vi "parseEngineeringStatus.vi"(8 "error in (no error)":errorcluster, 10 "engineeringStatusString":string, 11 "DomeCommunicator in":refnum<class "DomeCommunicator.lvclass">) -> (0 "error out":errorcluster, 2 "engineeringStatus":T1, 3 "DomeCommunicator out":refnum<class "DomeCommunicator.lvclass">)   [LabVIEW 2016, in "DomeCommunicator.lvclass"]
uses:
  DomeCommunicator.lvclass
  ComTypedefs/engineeringStatus.ctl
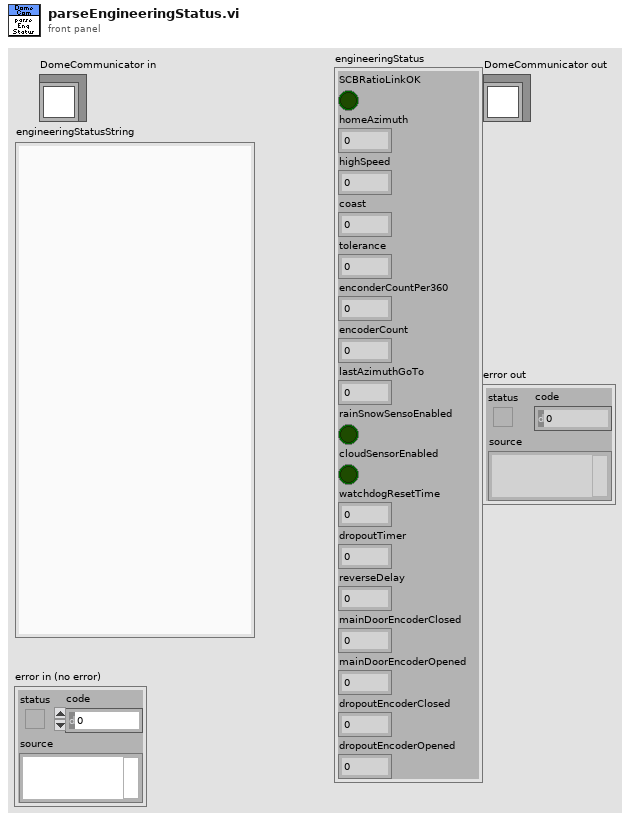
[diagram p1: front panel]
types:
  T1 = typedef "engineeringStatus.ctl" = cluster{"SCBRatioLinkOK":bool, "homeAzimuth":dbl, "highSpeed":dbl, "coast":dbl, "tolerance":dbl, "enconderCountPer360":u32, "encoderCount":u32, "lastAzimuthGoTo":dbl, "rainSnowSensoEnabled":bool, "cloudSensorEnabled":bool, "watchdogResetTime":dbl, "dropoutTimer":dbl, "reverseDelay":dbl, "mainDoorEncoderClosed":u32, "mainDoorEncoderOpened":u32, "dropoutEncoderClosed":u32, "dropoutEncoderOpened":u32}
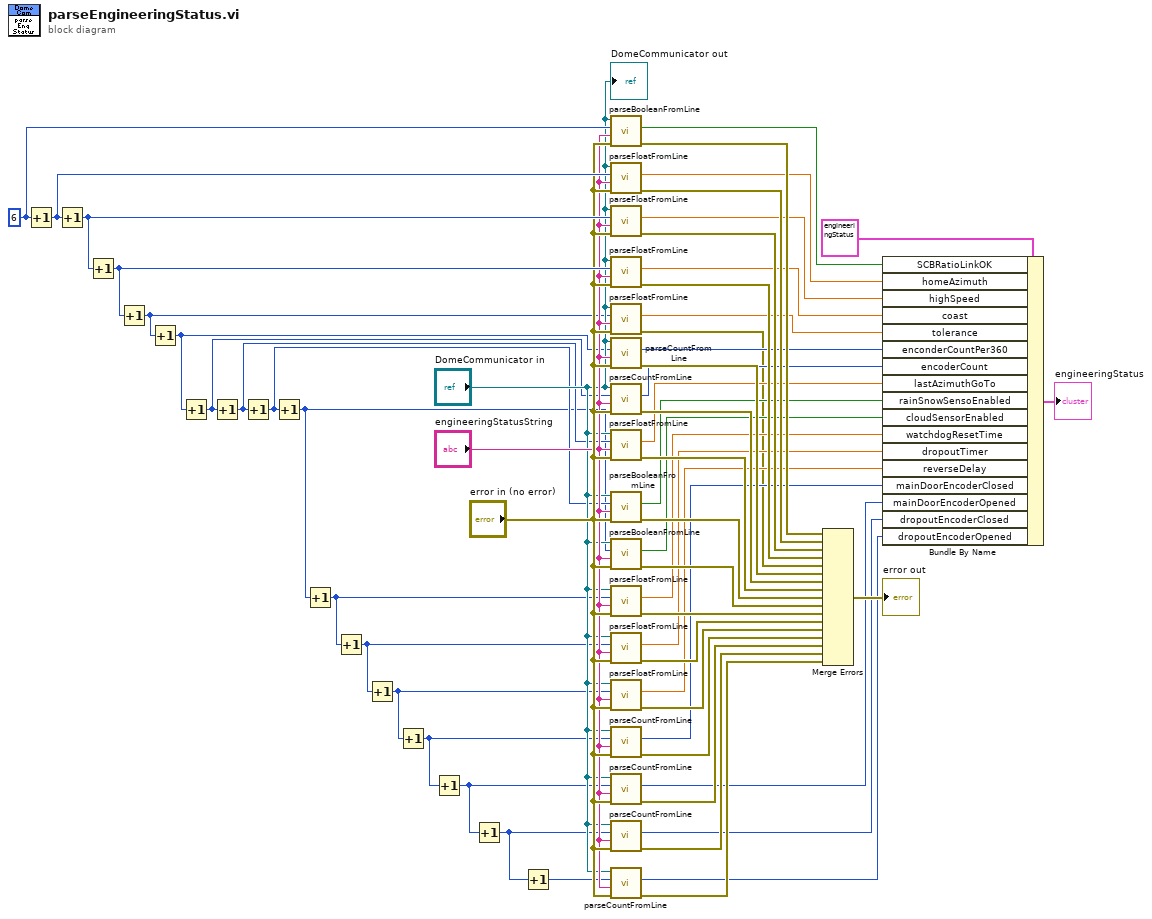
[diagram p0: block diagram]
diagram:
  w38 = u32 6 ("line")
  n1 = Increment(x=w38) -> (x+1=w37:u32)
  n2 = Increment(x=w37) -> (x+1=w36:u32)
  n3 = Increment(x=w36) -> (x+1=w35:u32)
  n4 = Increment(x=w35) -> (x+1=w13:u32)
  n5 = Increment(x=w13) -> (x+1=w12:u32)
  n6 = Increment(x=w12) -> (x+1=w11:u32)
  n7 = Increment(x=w11) -> (x+1=w10:u32)
  n8 = Increment(x=w10) -> (x+1=w9:u32)
  n9 = Increment(x=w9) -> (x+1=w8:u32)
  n10 = Increment(x=w8) -> (x+1=w7:u32)
  n11 = Increment(x=w7) -> (x+1=w6:u32)
  n12 = Increment(x=w6) -> (x+1=w5:u32)
  n13 = Increment(x=w5) -> (x+1=w4:u32)
  n14 = Increment(x=w4) -> (x+1=w3:u32)
  n15 = Increment(x=w3) -> (x+1=w2:u32)
  n16 = Increment(x=w2) -> (x+1=w1:u32)
  n17 = call "parseBooleanFromLine.vi"("error in (no error)"="error in (no error)", "engineeringStatus"="engineeringStatusString", "line"=w38, "DomeCommunicator in"="DomeCommunicator in") -> ("error out"=w55:errorcluster, "value"=w56:bool)  [unwired: 5 in, 1 out]
  n18 = call "parseFloatFromLine.vi"("error in (no error)"="error in (no error)", "engineeringStatus"="engineeringStatusString", "line"=w37, "DomeCommunicator in"="DomeCommunicator in") -> ("error out"=w54:errorcluster, "value"=w34:sgl)  [unwired: 5 in, 1 out]
  n19 = call "parseFloatFromLine.vi"("error in (no error)"="error in (no error)", "engineeringStatus"="engineeringStatusString", "line"=w36, "DomeCommunicator in"="DomeCommunicator in") -> ("error out"=w52:errorcluster, "value"=w33:sgl)  [unwired: 5 in, 1 out]
  n20 = call "parseFloatFromLine.vi"("error in (no error)"="error in (no error)", "engineeringStatus"="engineeringStatusString", "line"=w35, "DomeCommunicator in"="DomeCommunicator in") -> ("error out"=w51:errorcluster, "value"=w31:sgl)  [unwired: 5 in, 1 out]
  n21 = call "parseFloatFromLine.vi"("error in (no error)"="error in (no error)", "engineeringStatus"="engineeringStatusString", "line"=w13, "DomeCommunicator in"="DomeCommunicator in") -> ("error out"=w14:errorcluster, "value"=w27:sgl)  [unwired: 5 in, 1 out]
  n22 = call "parseCountFromLine.vi"("error in (no error)"="error in (no error)", "engineeringStatus"="engineeringStatusString", "line"=w12, "DomeCommunicator in"="DomeCommunicator in") -> ("error out"=w50:errorcluster, "value"=w26:u32)  [unwired: 5 in, 1 out]
  n23 = call "parseCountFromLine.vi"("error in (no error)"="error in (no error)", "engineeringStatus"="engineeringStatusString", "line"=w11, "DomeCommunicator in"="DomeCommunicator in") -> ("error out"=w49:errorcluster, "value"=w25:u32)  [unwired: 5 in, 1 out]
  n24 = call "parseFloatFromLine.vi"("error in (no error)"="error in (no error)", "engineeringStatus"="engineeringStatusString", "line"=w10, "DomeCommunicator in"="DomeCommunicator in") -> ("error out"=w48:errorcluster, "value"=w24:sgl)  [unwired: 5 in, 1 out]
  n25 = call "parseBooleanFromLine.vi"("error in (no error)"="error in (no error)", "engineeringStatus"="engineeringStatusString", "line"=w9, "DomeCommunicator in"="DomeCommunicator in") -> ("error out"=w47:errorcluster, "value"=w23:bool)  [unwired: 5 in, 1 out]
  n26 = call "parseBooleanFromLine.vi"("error in (no error)"="error in (no error)", "engineeringStatus"="engineeringStatusString", "line"=w8, "DomeCommunicator in"="DomeCommunicator in") -> ("error out"=w46:errorcluster, "value"=w22:bool)  [unwired: 5 in, 1 out]
  n27 = call "parseFloatFromLine.vi"("error in (no error)"="error in (no error)", "engineeringStatus"="engineeringStatusString", "line"=w7, "DomeCommunicator in"="DomeCommunicator in") -> ("error out"=w45:errorcluster, "value"=w21:sgl)  [unwired: 5 in, 1 out]
  n28 = call "parseFloatFromLine.vi"("error in (no error)"="error in (no error)", "engineeringStatus"="engineeringStatusString", "line"=w6, "DomeCommunicator in"="DomeCommunicator in") -> ("error out"=w44:errorcluster, "value"=w20:sgl)  [unwired: 5 in, 1 out]
  n29 = call "parseFloatFromLine.vi"("error in (no error)"="error in (no error)", "engineeringStatus"="engineeringStatusString", "line"=w5, "DomeCommunicator in"="DomeCommunicator in") -> ("error out"=w43:errorcluster, "value"=w19:sgl)  [unwired: 5 in, 1 out]
  n30 = call "parseCountFromLine.vi"("error in (no error)"="error in (no error)", "engineeringStatus"="engineeringStatusString", "line"=w4, "DomeCommunicator in"="DomeCommunicator in") -> ("error out"=w42:errorcluster, "value"=w18:u32)  [unwired: 5 in, 1 out]
  n31 = call "parseCountFromLine.vi"("error in (no error)"="error in (no error)", "engineeringStatus"="engineeringStatusString", "line"=w3, "DomeCommunicator in"="DomeCommunicator in") -> ("error out"=w41:errorcluster, "value"=w17:u32)  [unwired: 5 in, 1 out]
  n32 = call "parseCountFromLine.vi"("error in (no error)"="error in (no error)", "engineeringStatus"="engineeringStatusString", "line"=w2, "DomeCommunicator in"="DomeCommunicator in") -> ("error out"=w40:errorcluster, "value"=w16:u32)  [unwired: 5 in, 1 out]
  n33 = call "parseCountFromLine.vi"("error in (no error)"="error in (no error)", "engineeringStatus"="engineeringStatusString", "line"=w1, "DomeCommunicator in"="DomeCommunicator in") -> ("error out"=w39:errorcluster, "value"=w15:u32)  [unwired: 5 in, 1 out]
  n34 = Merge Errors(w55, w54, w52, w51, w14, w50, w49, w48, w47, w46, w45, w44, w43, w42, w41, w40, w39) -> (→"error out":errorcluster)
  n35 = Bundle By Name(cluster=T1 {"SCBRatioLinkOK"=FALSE, "homeAzimuth"=0.0, "highSpeed"=0.0, "coast"=0.0, "tolerance"=0.0, "enconderCountPer360"=0, "encoderCount"=0, "lastAzimuthGoTo"=0.0, "rainSnowSensoEnabled"=FALSE, "cloudSensorEnabled"=FALSE, "watchdogResetTime"=0.0, "dropoutTimer"=0.0, "reverseDelay"=0.0, "mainDoorEncoderClosed"=0, "mainDoorEncoderOpened"=0, "dropoutEncoderClosed"=0, "dropoutEncoderOpened"=0} ("engineeringStatus"), "SCBRatioLinkOK"=w56, "homeAzimuth"=w34, "highSpeed"=w33, "coast"=w31, "tolerance"=w27, "enconderCountPer360"=w26, "encoderCount"=w25, "lastAzimuthGoTo"=w24, "rainSnowSensoEnabled"=w23, "cloudSensorEnabled"=w22, "watchdogResetTime"=w21, "dropoutTimer"=w20, "reverseDelay"=w19, "mainDoorEncoderClosed"=w18, "mainDoorEncoderOpened"=w17, "dropoutEncoderClosed"=w16, "dropoutEncoderOpened"=w15) -> (→"engineeringStatus":T1)
  "DomeCommunicator out" <- "DomeCommunicator in"
